vi "TDT-Get Artifact Times.vi"(0 "Data":T1={"TTankX"=refnum, "TDevAccX"=refnum, "LastTime"=0.0, "error"={"status"=FALSE, "code"=0, "source"=""}, "Block Name"="", "Circuit Tag"="", "Tank Name"="", "NumTicks"=0, "LastTick"=0.0, "Idle?"=FALSE, "Wait (ms)"=1000, "LastArtf"=0.0, "LastTosc"=0.0}, 5 "T2":dbl, 7 "Max Read":i32=1000, 11 "error in (no error)":errorcluster) -> (6 "Number of Artifacts":i32, 8 "Artifact Times":dbl[][](array[numeric]), 15 "error out":errorcluster)   [LabVIEW 2015]
uses:
  TDT Interface Data.ctl
panel:
  out "Numeric":i32
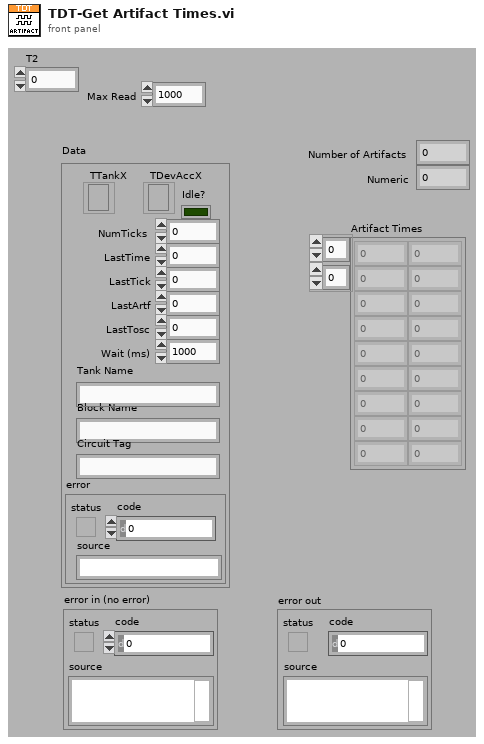
[diagram p1: front panel]
types:
  T1 = typedef "TDT Interface Data.ctl" = cluster{"TTankX":refnum<k7>, "TDevAccX":refnum<k7>, "LastTime":dbl, "error":errorcluster, "Block Name":string, "Circuit Tag":string, "Tank Name":string, "NumTicks":i32, "LastTick":dbl, "Idle?":bool, "Wait (ms)":u32, "LastArtf":dbl, "LastTosc":dbl}
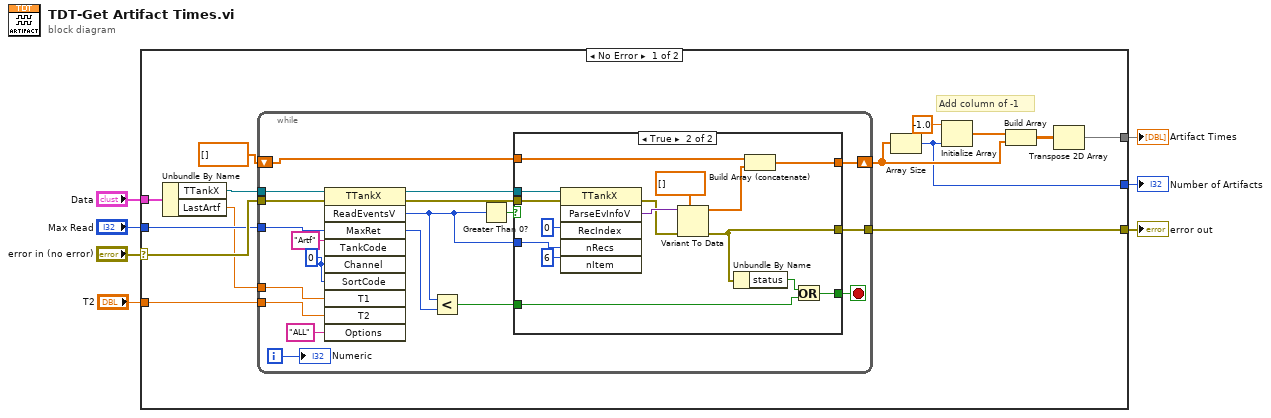
[diagram p0: block diagram]
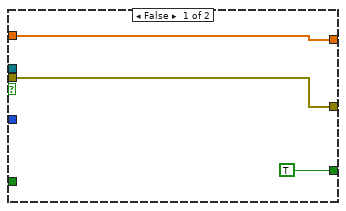
[diagram p2: hidden frame]
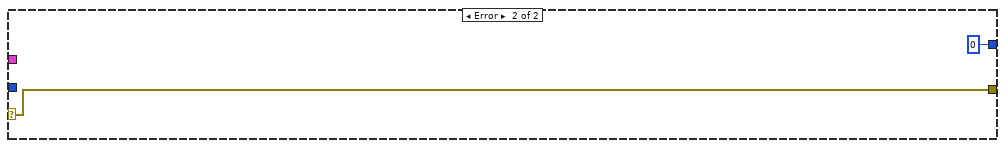
[diagram p3: hidden frame]
diagram:
  n1 = case shown="No Error" "error in (no error)" {
    selector: "error in (no error)" -> [w19 w60]
    tunnel: "Data" -> [w21 _]
    tunnel: "Max Read" -> [w18 _]
    tunnel: [w15 w60] -> w4
    tunnel: [w10 _] -> w3
    tunnel: [w9 0] -> w2
    tunnel: "T2" -> [w8 _]
    frame No Error {
      # "Add column of -1"
      n2 = Unbundle By Name(w21) -> ("TTankX"=w20:refnum<k7>, "LastArtf"=w17:dbl)
      n3 = while {
        tunnel: w20 -> [w40]
        tunnel: w19 -> [w39]
        tunnel: w18 -> [w38]
        tunnel: w17 -> [w37]
        shift-right: [w28] -> w12
        shift-left: dbl[] [] -> [w27]
        tunnel: [w26] -> w15
        tunnel: w8 -> [w22]
        i -> [w23]
        stop <- w32 stop-if-true
        w35 = 0 ("Channel")
        n4 = invoke class="TTankX" method="ReadEventsV"(reference=w40, error in=w39, "MaxRet"=w38, "TankCode"="Artf", "Channel"=w35, "SortCode"=w35, "T1"=w37, "T2"=w22, "Options"="ALL") -> (reference out=w30:refnum<k7>, error out=w29:errorcluster, "ReadEventsV"=w24:i32, "MaxRet"=w33:i32)  [unwired: 1 in, 6 out]
        n5 = Less?(x=w24, y=w33) -> (x < y?=w31:bool)
        n6 = Greater Than 0?(x=w24) -> (x > 0?=w25:bool)
        n7 = case shown="True" w25 {
          tunnel: [TRUE w58] -> w32
          tunnel: w31 -> [_ w56]
          tunnel: w30 -> [_ w55]
          tunnel: w29 -> [w42 w54]
          tunnel: w24 -> [_ w52]
          tunnel: [w43 w46] -> w28
          tunnel: w27 -> [w43 w45]
          tunnel: [w42 w44] -> w26
          frame False {
          }
          frame True {
            n8 = invoke class="TTankX" method="ParseEvInfoV"(reference=w55, error in=w54, "RecIndex"=0, "nRecs"=w52, "nItem"=6) -> (error out=w48:errorcluster, "ParseEvInfoV"=w50:variant)  [unwired: 1 in, 4 out]
            n9 = Variant To Data(error in=w48, type=dbl[] [], Variant=w50) -> (data=w47:dbl[], error out=w44:errorcluster)
            n10 = Unbundle By Name(w44) -> ("status"=w57:bool)
            n11 = Build Array (concatenate)(w45, w47) -> (w46:dbl[])
            n12 = Or(x=w57, y=w56) -> (x .or. y?=w58:bool)
          }
        }
        "Numeric" <- w23
      }
      n13 = Array Size(array=w12) -> (size(s)=w9:i32)
      n14 = Initialize Array(-1.0 ("element"), w9) -> (w13:dbl[])
      n15 = Build Array(w13, w12) -> (w11:dbl[][])
      n16 = Transpose 2D Array(2D array=w11) -> (transposed array=w10:dbl[][])
    }
    frame Error {
    }
  }
  "Artifact Times" <- w3
  "error out" <- w4
  "Number of Artifacts" <- w2
